vi "Z900_navX_Util_LittleEndian_to_BigEndian.vi"(1 "Little Endian":u8[](array[numeric])) -> (0 "Big Endian":u8[](array[numeric]))   [LabVIEW 2019]
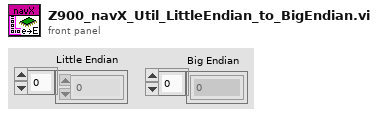
[diagram p1: front panel]
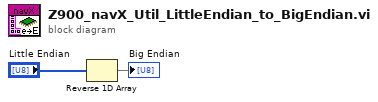
[diagram p0: block diagram]
diagram:
  n1 = Reverse 1D Array(array="Little Endian") -> (reversed array=→"Big Endian":u8[])
